vi "A170316-11-Login.vi"() -> ()   [LabVIEW 2020]
uses:
  Database/Global1.vi
  <vilib>/addons/database/Connection.llb/DB Tools Open Connec (String).vi
  <vilib>/addons/database/Connection.llb/Conn Execute.vi
  <vilib>/addons/database/Recordset.llb/Rec Fetch Recordset Data (R).vi
  <vilib>/addons/database/NI_Database_API.lvlib
  <vilib>/addons/database/Recordset.llb/Rec Destroy - Connection.vi
panel:
  in  "登陆":bool
  in  "密   码":string
  out "数据库连接成功":bool
  in  "联机模式":enum16{"单机", "联网"}(ring)
  in  "用户名":string
  # "数据库状态"
  # "激光打标机"
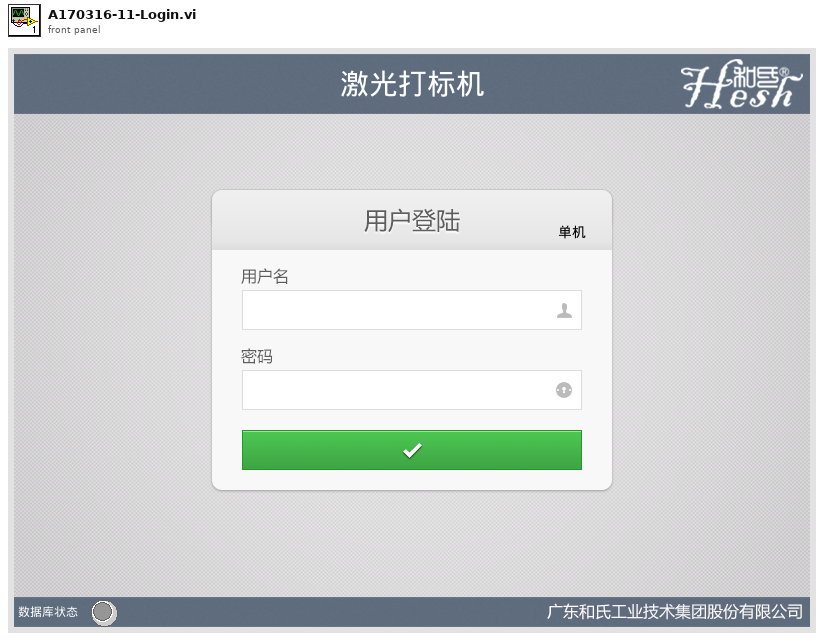
[diagram p1: front panel]
types:
  T1 = enum8{"Enabled", "Disabled", "Disabled and Grayed Out"}
  T2 = enum32{"Invalid", "Standard", "Closed", "Hidden", "Minimized", "Maximized"}
  T3 = cluster{"data[0]":string, "data[1]":string, "data[2]":string, "data[3]":string}
  T4 = typedef "NI_Database_API.lvlib/Conn ObjectReference.ctl" = refnum<k1>
  T5 = typedef "NI_Database_API.lvlib/Rec ObjectReference.ctl" = refnum<k1>
  T6 = typedef "eventvkey.ctl" = enum16{"ASCII", "Enter", "Return", "Shift", "Ctrl", "Alt", "Cmd", "Opt", "Caps", "NumLock", "Clear", "Break", "Up", "Down", "Left", "Right", "Insert", "Delete", "Home", "End", "PageUp", "PageDown", "Escape", "Help", "Pause", "ScrollLock", "F1", "F2", "F3", "F4", "F5", "F6", "F7", "F8", "F9", "F10", "F11", "F12", "F13", "F14", "F15", "F16", "F17", "F18", "F19", "F20", "F21", "F22", "F23", "F24", "Play", "VolumeUp", "VolumeDown", "Mute", "Two Byte Char"}
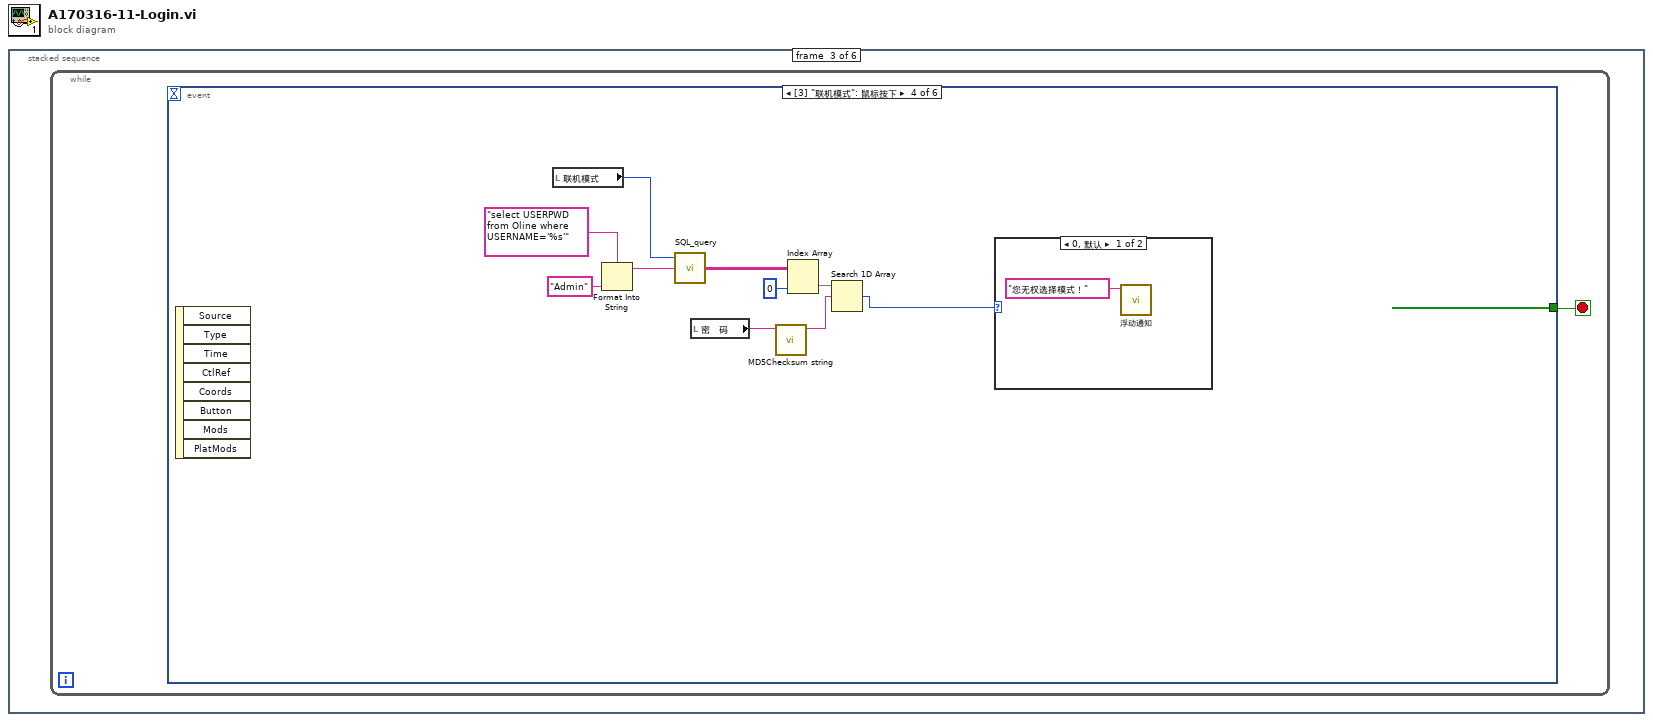
[diagram p0: block diagram]
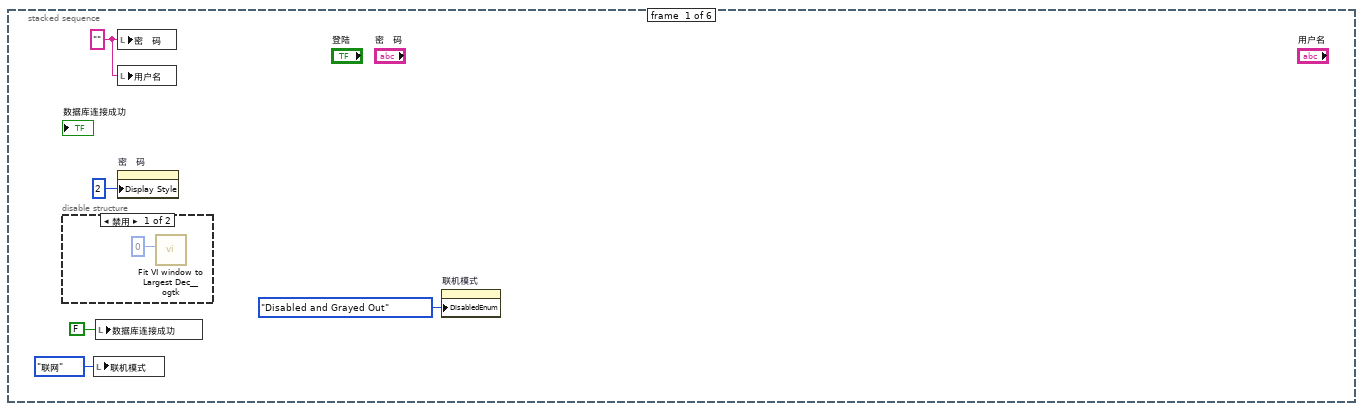
[diagram p2: hidden frame]
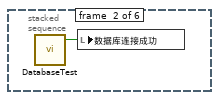
[diagram p4: hidden frame]
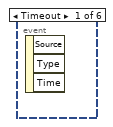
[diagram p5: hidden frame]
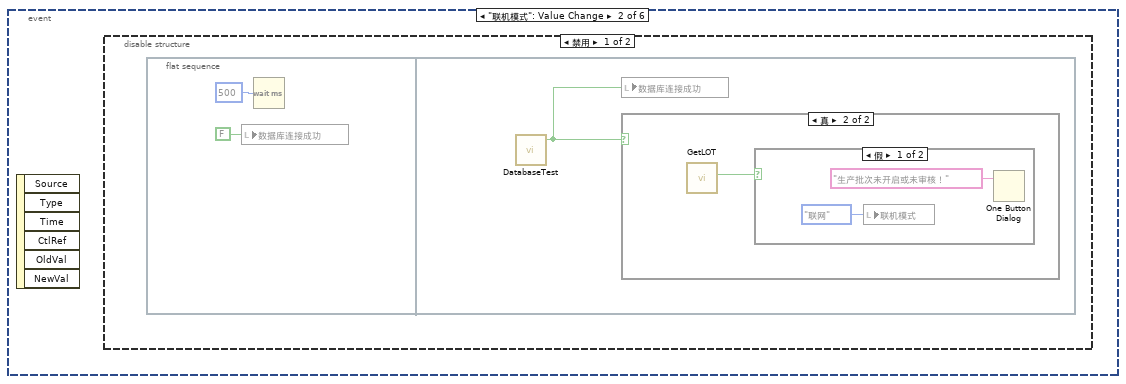
[diagram p6: hidden frame]
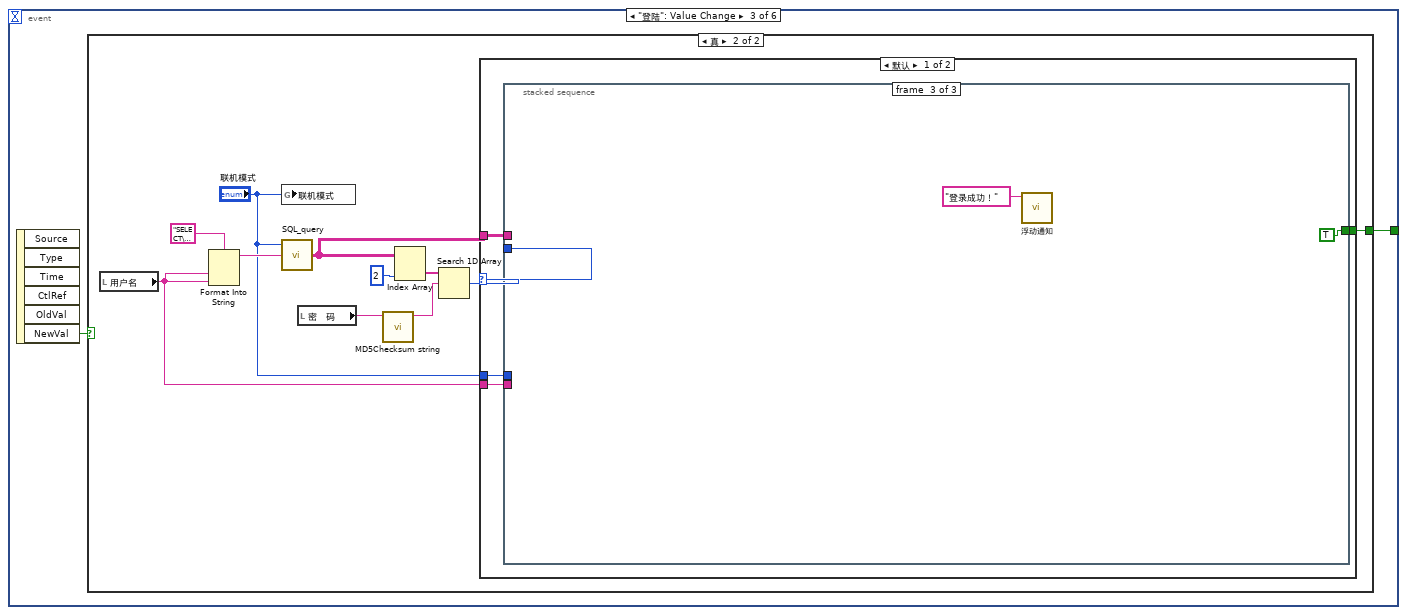
[diagram p10: hidden frame]
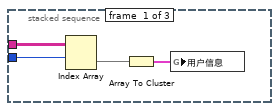
[diagram p12: hidden frame]
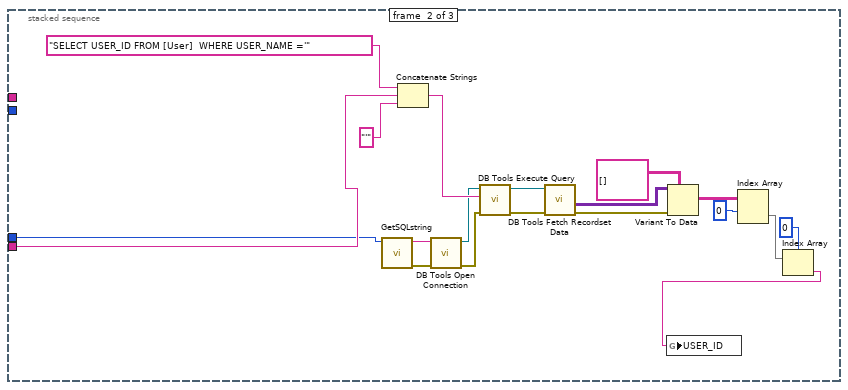
[diagram p13: hidden frame]
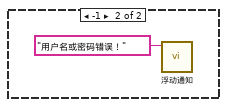
[diagram p14: hidden frame]
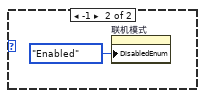
[diagram p15: hidden frame]
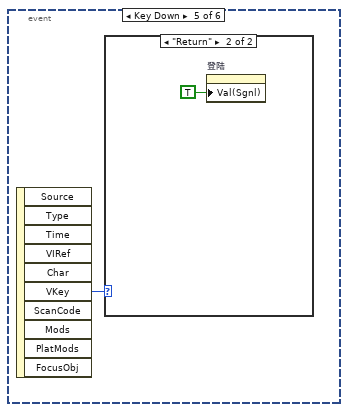
[diagram p16: hidden frame]
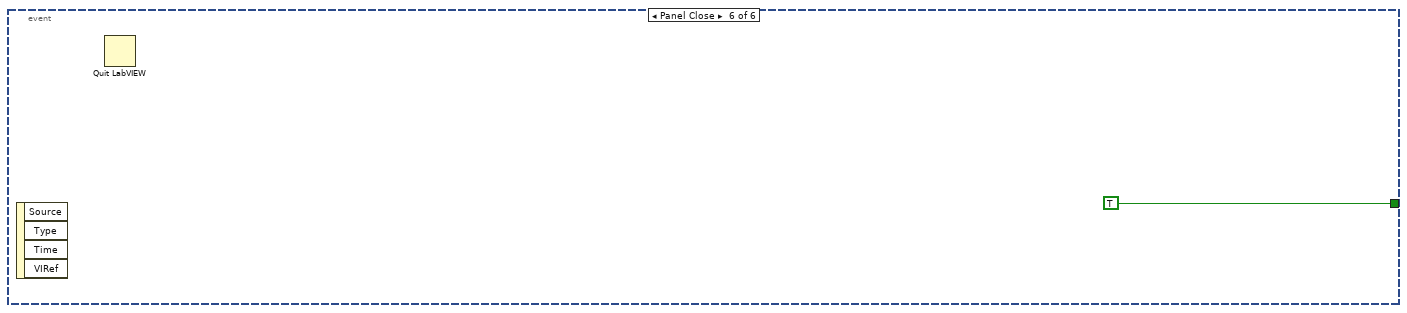
[diagram p18: hidden frame]
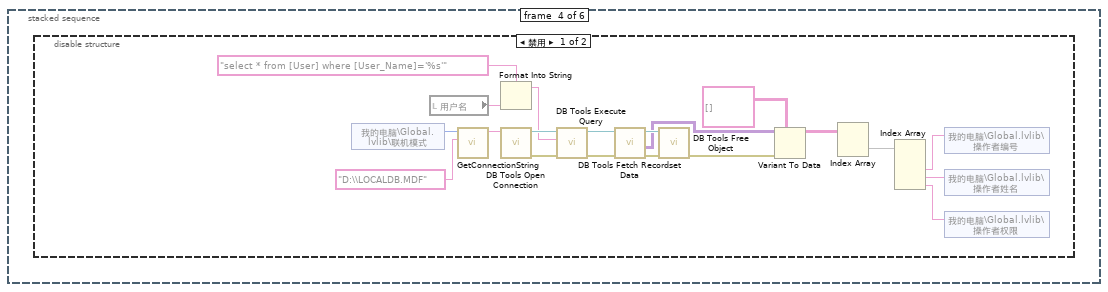
[diagram p19: hidden frame]
diagram:
  n1 = stacked-sequence {
    frame #0 {
      w4 = ""
      n2 = disable-structure shown="禁用" {
        frame Disabled {
          n3 = call <userlib>:"Fit VI window to Largest Dec__ogtk.vi"("border spacing (2 px)"=0) -> ()  [unwired: 5 in, 2 out]
        }
        frame Enabled {
        }
      }
      n4 = local write "联机模式"(enum16{"单机", "联网"}."联网" ("联机模式")) -> ()
      n5 = local write "数据库连接成功"(FALSE ("数据库连接成功")) -> ()
      n6 = local write "密   码"(w4) -> ()
      n7 = local write "用户名"(w4) -> ()
      n8 = property on="密   码" class="Str"("Display Style"=u32 2 ("显示样式")) -> ()  [unwired: 2 in, 2 out]
      n9 = property on="联机模式" class="Enum (严格)"("DisabledEnum"=T1."Disabled and Grayed Out" ("禁用")) -> ()  [unwired: 2 in, 2 out]
    }
    frame #1 {
      n10 = call "DatabaseTest.vi"() -> ("数据库连接成功"=w7:bool)  [unwired: 4 in, 1 out]
      n11 = local write "数据库连接成功"(w7) -> ()
    }
    frame #2 {
      n12 = while {
        stop <- w8 stop-if-true
        n13 = event shown="[3] \"联机模式\": 鼠标按下" {
          selector: _ -> [_ _ _ _ _ _]
          dyn-events: _ -> [_ _ _ _ _ _]
          timeout: _ -> [_ _ _ _ _ _]
          tunnel: [_ _ w15 _ _ TRUE] -> w8
          event Timeout {
            n14 = event-data() -> ()  [unwired: 1 in, 3 out]
          }
          event "联机模式": Value Change {
            n15 = event-data() -> ()  [unwired: 1 in, 6 out]
            n16 = disable-structure shown="禁用" {
              frame Disabled {
                n17 = flat-sequence {
                  frame #0 {
                    n18 = local write "数据库连接成功"(FALSE ("数据库连接成功")) -> ()
                    n19 = Wait (ms)(milliseconds to wait=u32 500 ("等待时间（毫秒）")) -> ()  [unwired: 1 out]
                  }
                  frame #1 {
                    n20 = call "DatabaseTest.vi"() -> ("数据库连接成功"=w11:bool)  [unwired: 4 in, 1 out]
                    n21 = local write "数据库连接成功"(w11) -> ()
                    n22 = case shown="真" w11 {
                      frame False {
                      }
                      frame True {
                        n23 = call "GetLOT.vi"() -> ("生产批次有效"=w12:bool)  [unwired: 9 in, 2 out]
                        n24 = case shown="假" w12 {
                          frame False {
                            n25 = local write "联机模式"(enum16{"单机", "联网"}."联网" ("联机模式")) -> ()
                            n26 = One Button Dialog(message="生产批次未开启或未审核！" ("消息")) -> ()  [unwired: 1 in, 1 out]
                          }
                          frame True {
                          }
                        }
                      }
                    }
                  }
                }
              }
              frame Enabled {
              }
            }
          }
          event "登陆": Value Change {
            n27 = event-data() -> ("NewVal"=w16:bool)  [unwired: 1 in, 5 out]
            n28 = case shown="真" w16 {
              tunnel: [_ w19] -> w15
              frame False {
              }
              frame True {
                n29 = local read "用户名"() -> (w18:string)
                n30 = Format Into String(format string="SELECT\ndbo.[User].USER_EMPLOYEE_ID,\ndbo.[User].USER_NAME,\ndbo.[User].USER_PASSWD,\ndbo.[User].USER_PERMIT\n\nFROM\ndbo.[User]\nWHERE\ndbo.[User].USER_NAME = '%s' \nOR\ndbo.[User].USER_EMPLOYEE_ID = '%s'\n" ("格式字符串"), w18, w18) -> (resulting string=w25:string)  [unwired: 2 in, 1 out]
                n31 = global write "Global1.vi" "联机模式"("联机模式") -> ()
                n32 = call "SQL_query.vi"("SQL query"=w25, "联机模式"="联机模式") -> ("data"=w20:string[][])  [unwired: 1 in, 2 out]
                n33 = local read "密   码"() -> (w27:string)
                n34 = call <vilib>:"MD5Checksum string.vi"("Message String"=w27) -> ("MD5 message-digest"=w21:string)  [unwired: 10 in]
                n35 = Index Array(array=w20, index (col)=2 ("禁用的索引 (列)")) -> (element=w24:string[])  [unwired: 1 in]
                n36 = Search 1D Array(1D array=w24, element=w21) -> (index of element=w22:i32)  [unwired: 1 in]
                n37 = case shown="默认" w22 {
                  selector: w22 -> [w32 _]
                  tunnel: w20 -> [w31 _]
                  tunnel: [w30 _] -> w19
                  tunnel: w18 -> [w29 _]
                  tunnel: "联机模式" -> [w28 _]
                  frame Default {
                    n38 = stacked-sequence {
                      tunnel: w32 -> [w33 _ _]
                      tunnel: w31 -> [w35 _ _]
                      tunnel: [_ _ TRUE] -> w30
                      tunnel: w29 -> [_ w39 _]
                      tunnel: w28 -> [_ w38 _]
                      frame #0 {
                        n39 = Index Array(array=w35, index (row)=w33) -> (element=w34:string[])  [unwired: 1 in]
                        n40 = Array To Cluster(array=w34) -> (cluster=w36:T3)
                        n41 = global write "Global1.vi" "用户信息"(w36) -> ()
                      }
                      frame #1 {
                        n42 = call "GetSQLstring.vi"("联机模式"=w38) -> ("错误输出"=w54:errorcluster, "连接字符串"=w55:string)  [unwired: 9 in]
                        n43 = Concatenate Strings("SELECT USER_ID FROM [User]  WHERE USER_NAME ='" ("字符串"), w39, "'" ("字符串")) -> (w53:string)
                        n44 = call-poly <vilib>:"DB Tools Open Connection.vi"("error in (no error)"=w54, "connection information"=w55) -> ("error out"=w47:errorcluster, "connection reference"=w48:T4)  [unwired: 6 in]
                        n45 = call-poly <vilib>:"DB Tools Execute Query.vi"("error in (no error)"=w47, "SQL query"=w53, "connection reference"=w48) -> ("error out"=w51:errorcluster, "recordset reference"=w52:T5)  [unwired: 5 in]
                        n46 = call-poly <vilib>:"DB Tools Fetch Recordset Data.vi"("error in (no error)"=w51, "recordset reference"=w52) -> ("error out"=w45:errorcluster, "recordset data"=w50:variant[][])  [unwired: 3 in, 1 out]
                        n47 = Variant To Data(error in=w45, type=string[][] [], Variant=w50) -> (data=w44:string[][])  [unwired: 1 out]
                        n48 = Index Array(array=w44, index (row)=0 ("索引 (行)")) -> (element=w42:string[])  [unwired: 1 in]
                        n49 = Index Array(array=w42, index=0 ("索引 (行)")) -> (element=w37:string)
                        n50 = global write "Global1.vi" "USER_ID"(w37) -> ()
                      }
                      frame #2 {
                        n51 = call "浮动通知.vi"("通知内容"="登录成功！") -> ()  [unwired: 11 in]
                      }
                    }
                  }
                  frame -1 {
                    n52 = call "浮动通知.vi"("通知内容"="用户名或密码错误！") -> ()  [unwired: 11 in]
                  }
                }
              }
            }
          }
          event "联机模式": Mouse Down {
            n53 = event-data() -> ()  [unwired: 1 in, 8 out]
            n54 = local read "联机模式"() -> (w61:enum16{"单机", "联网"})
            n55 = Format Into String(format string="select USERPWD from Oline where USERNAME='%s'" ("格式字符串"), "Admin" ("输入 1")) -> (resulting string=w67:string)  [unwired: 2 in, 1 out]
            n56 = call "SQL_query.vi"("SQL query"=w67, "联机模式"=w61) -> ("data"=w64:string[][])  [unwired: 1 in, 2 out]
            n57 = local read "密   码"() -> (w68:string)
            n58 = call <vilib>:"MD5Checksum string.vi"("Message String"=w68) -> ("MD5 message-digest"=w65:string)  [unwired: 10 in]
            n59 = Index Array(array=w64, index (col)=0 ("禁用的索引 (列)")) -> (element=w66:string[])  [unwired: 1 in]
            n60 = Search 1D Array(1D array=w66, element=w65) -> (index of element=w59:i32)  [unwired: 1 in]
            n61 = case shown="0, 默认" w59 {
              frame 0, Default {
                n62 = call "浮动通知.vi"("通知内容"="您无权选择模式！") -> ()  [unwired: 11 in]
              }
              frame -1 {
                n63 = property on="联机模式" class="Enum (严格)"("DisabledEnum"=T1."Enabled" ("禁用")) -> ()  [unwired: 2 in, 2 out]
              }
            }
          }
          event Key Down {
            n64 = event-data() -> ("VKey"=w71:T6)  [unwired: 1 in, 9 out]
            n65 = case shown="\"Return\"" w71 {
              frame "ASCII", Default {
              }
              frame "Return" {
                n66 = property on="登陆" class="Bool (严格)"("Val(Sgnl)"=TRUE ("值(信号)")) -> ()  [unwired: 2 in, 2 out]
              }
            }
          }
          event Panel Close {
            n67 = event-data() -> ()  [unwired: 1 in, 4 out]
            n68 = Quit LabVIEW() -> ()  [unwired: 1 in]
          }
        }
      }
    }
    frame #3 {
      n69 = disable-structure shown="禁用" {
        frame Disabled {
          n70 = shared-variable "我的电脑\\Global.lvlib\\联机模式"() -> (w74:i16)  [unwired: 1 in, 1 out]
          n71 = local read "用户名"() -> (w76:string)
          n72 = call "GetConnectionString.vi"("Database Name"="D:\\LOCALDB.MDF", "连接模式"=w74) -> ("连接字符串"=w92:string)  [unwired: 4 in, 1 out]
          n73 = Format Into String(format string="select * from [User] where [User_Name]='%s'", w76) -> (resulting string=w75:string)  [unwired: 2 in, 1 out]
          n74 = call-poly <vilib>:"DB Tools Open Connection.vi"("connection information"=w92) -> ("error out"=w91:errorcluster, "connection reference"=w90:T4)  [unwired: 7 in]
          n75 = call-poly <vilib>:"DB Tools Execute Query.vi"("error in (no error)"=w91, "SQL query"=w75, "connection reference"=w90) -> ("error out"=w87:errorcluster, "recordset reference"=w89:T5)  [unwired: 5 in]
          n76 = call-poly <vilib>:"DB Tools Fetch Recordset Data.vi"("error in (no error)"=w87, "recordset reference"=w89) -> ("error out"=w86:errorcluster, "recordset data"=w84:variant[][], "recordset reference out"=w88:T5)  [unwired: 3 in]
          n77 = call-poly <vilib>:"DB Tools Free Object.vi"("error in (no error)"=w86, "recordset reference"=w88) -> ("error out"=w85:errorcluster)  [unwired: 8 in, 1 out]
          n78 = Variant To Data(error in=w85, type=string[][] [], Variant=w84) -> (data=w82:string[][])  [unwired: 1 out]
          n79 = Index Array(array=w82) -> (element=w81:string[])  [unwired: 2 in]
          n80 = Index Array(array=w81) -> (element #2=w78:string, element #3=w79:string, element #4=w80:string)  [unwired: 4 in, 1 out]
          n81 = shared-variable "我的电脑\\Global.lvlib\\操作者编号"(w78) -> ()  [unwired: 1 in, 1 out]
          n82 = shared-variable "我的电脑\\Global.lvlib\\操作者姓名"(w79) -> ()  [unwired: 1 in, 1 out]
          n83 = shared-variable "我的电脑\\Global.lvlib\\操作者权限"(w80) -> ()  [unwired: 1 in, 1 out]
        }
        frame Enabled {
        }
      }
    }
    frame #4 {
      n84 = vi-ref "A170316-11-Main-large.vi"() -> (w95:refnum<vi>)
      n85 = call "CallVI.vi"("VI引用"=w95, "状态"=T2."Maximized") -> ()  [unwired: 11 in, 3 out]
    }
    frame #5 {
      n86 = control-ref of="本VI"() -> (w96:refnum<vi>)
      n87 = invoke class="VI" method="FP.Close"(reference=w96) -> (reference out=w97:refnum<vi>, error out=w98:errorcluster)  [unwired: 2 in, 1 out]
      n88 = Close Reference(reference=w97, error in (no error)=w98) -> ()  [unwired: 1 out]
    }
  }
